vi "Tape Sensor (Sub VI).vi"() -> (1 "Edge":bool, 3 "Position To Add 1":dbl)   [LabVIEW 2017]
uses:
  <vilib>/functionblocks/Edge Detection/Edge Detect/Edge Detect.vi
  <vilib>/functionblocks/FB Core/FB Core.xnode
  <vilib>/functionblocks/NI_FunctionBlock Libraries.lvlib
panel:
  out "Waveform Chart":dbl(graph)
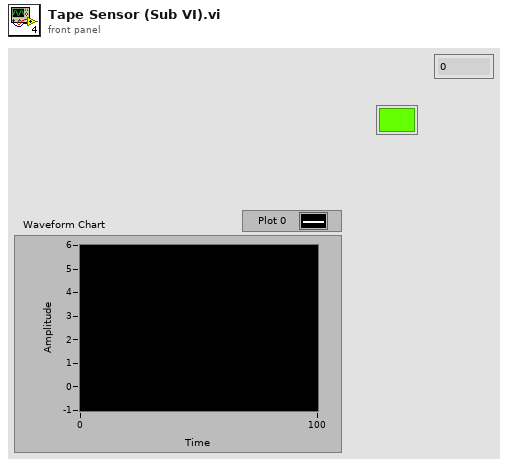
[diagram p1: front panel]
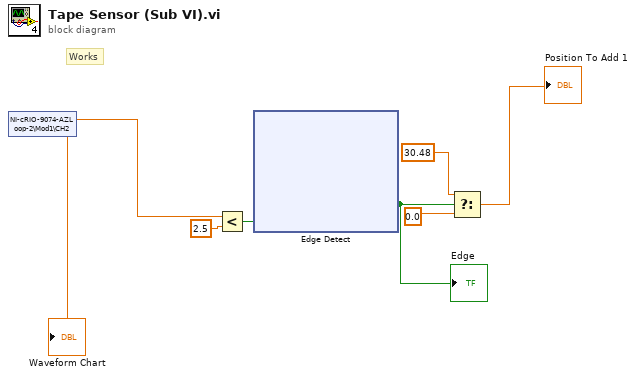
[diagram p0: block diagram]
diagram:
  # "Works"
  n1 = shared-variable "NI-cRIO-9074-AZLoop-2\\Mod1\\CH2"() -> (w1:dbl)  [unwired: 1 in, 1 out]
  "Waveform Chart" <- w1
  n2 = Less?(x=w1, y=2.5) -> (x < y?=w6:bool)
  n3 = xnode "Edge Detect"("input 1"=w6) -> ("output"=w2:bool)  [unwired: 2 in, 1 out]
  "Edge" <- w2
  n4 = Select(t=30.48, s=w2, f=0.0) -> (s? t:f=→"Position To Add 1":dbl)
